vi "ISX3_Cmd_GetSetupFrequencyPoint.vi"(1 "Row":u16=1 min=1 max=2048) -> (0 "get Setup Frequency Point Cmd":u8[](array[numeric]))   [LabVIEW 2012, in "Sciospec ISX3 Impedance Analyzer.lvlib"]
uses:
  Sciospec ISX3 Impedance Analyzer.lvlib
panel:
  # "This VI generates the command to read one line of a configured setup."
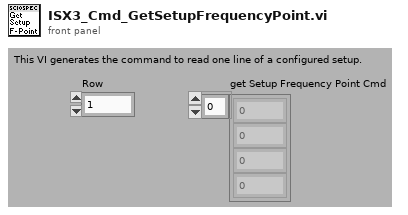
[diagram p1: front panel]
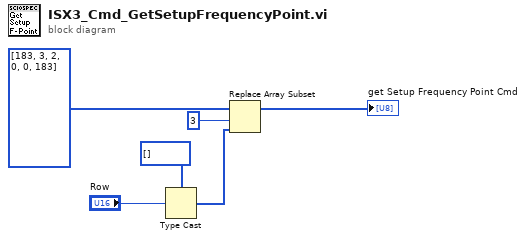
[diagram p0: block diagram]
diagram:
  n1 = Type Cast(type=u8[] [], x="Row") -> (*(type *) &x=w2:u8[])
  n2 = Replace Array Subset(array=u8[] [183, 3, 2, 0, 0, 183], new element=w2, index=3) -> (→"get Setup Frequency Point Cmd":u8[])
